vi "TEST PICOSCOPE 3000.vi"() -> ()   [LabVIEW 2018]
panel:
  in  "Acquisition Settings":T1={"preTriggerSamples"=0, "postTriggerSamples"=10000, "timebase"=5000, "Down-Sample Mode"=0, "Down Sample Ratio"=1} {"Down Sample Ratio" min=1 step=1; "Down-Sample Mode" items=["None"=0, "Aggregate"=1, "Decimate"=2, "Average"=4]; "postTriggerSamples" max=10000 step=100}
  out "Device Info":T2
  in  "Channel B Settings":T3={"Enabled"=TRUE, "Coupling"=1, "Range"=6, "Analogue Offset"=0.0} {"Range" items=["20 mV"=1, "50 mV"=2, "100 mV"=3, "200 mV"=4, "500 mV"=5, "1 V"=6, "2 V"=7, "5 V"=8, "10 V"=9, "20 V"=10]; "Coupling" items=["AC", "DC"]}
  in  "Channel A Settings":T3={"Enabled"=TRUE, "Coupling"=1, "Range"=6, "Analogue Offset"=0.0} {"Range" items=["20 mV"=1, "50 mV"=2, "100 mV"=3, "200 mV"=4, "500 mV"=5, "1 V"=6, "2 V"=7, "5 V"=8, "10 V"=9, "20 V"=10]; "Coupling" items=["AC", "DC"]}
  out "Waveform Graph 2":T4(graph)
  out "Waveform Graph":T4(graph)
  in  "Trigger Settings":T5={"Trigger Enabled"=TRUE, "Trigger Source"=enum."Channel A", "Trigger Threshold (Volts)"=0.0, "Trigger Direction"=2, "Trigger Delay (samples)"=0, "Auto Trigger Time (ms)"=1000} {"Trigger Direction" items=["Rising"=2, "Falling"=3]}
  # "127"
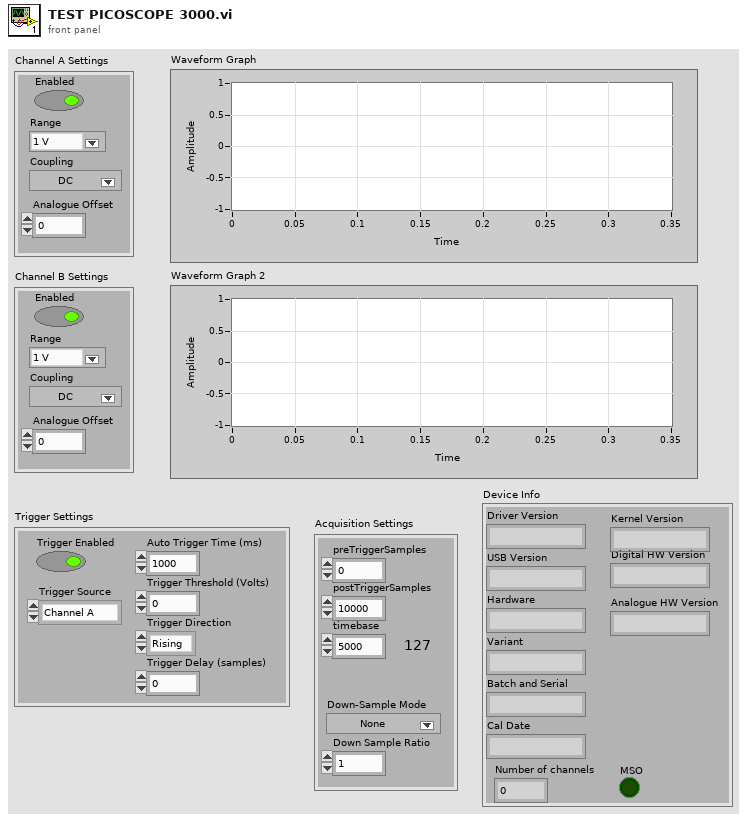
[diagram p1: front panel]
types:
  T1 = cluster{"preTriggerSamples":u32, "postTriggerSamples":u32, "timebase":u32, "Down-Sample Mode":i32, "Down Sample Ratio":u32}
  T2 = cluster{"Driver Version":string, "USB Version":string, "Hardware":string, "Variant":string, "Batch and Serial":string, "Cal Date":string, "Kernel Version":string, "Digital HW Version":string, "Analogue HW Version":string, "MSO":bool, "Number of channels":i16}
  T3 = cluster{"Enabled":bool, "Coupling":i16, "Range":u16, "Analogue Offset":sgl}
  T4 = cluster{i32, "Sample Internal":sgl, "Data (Volts)":dbl[]}
  T5 = cluster{"Trigger Enabled":bool, "Trigger Source":enum16{"Channel A", "Channel B", "Channel C", "Channel D", "Ext."}, "Trigger Threshold (Volts)":dbl, "Trigger Direction":u16, "Trigger Delay (samples)":u32, "Auto Trigger Time (ms)":i16}
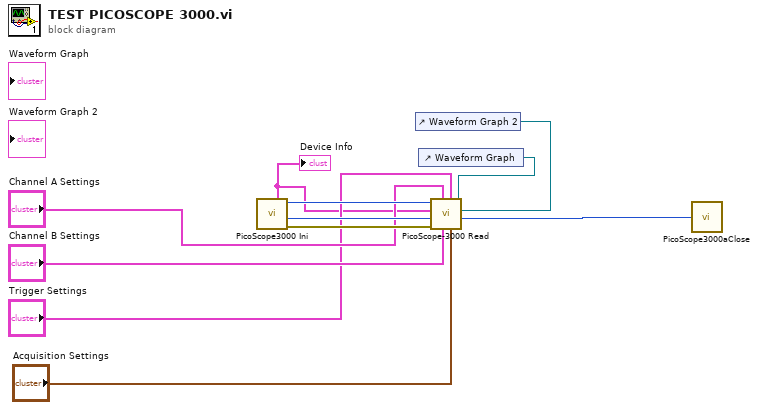
[diagram p0: block diagram]
diagram:
  n1 = call "PicoScope3000 Ini.vi"() -> ("error out"=w6:errorcluster, "Max Adc value"=w7:i16, "handle"=w11:i16, "Device Info"=w1:T2)  [unwired: 6 in, 2 out]
  "Device Info" <- w1
  n2 = control-ref of="Waveform Graph 2"() -> (w8:refnum<vi>)
  n3 = control-ref of="Waveform Graph"() -> (w9:refnum<vi>)
  n4 = call "PicoScope-3000 Read.vi"("WFD-Ref Ch-B"=w8, "WFD-Ref Ch-A"=w9, "Acquisition Settings"="Acquisition Settings", "Trigger Settings"="Trigger Settings", "Channel B Settings"="Channel B Settings", "Channel A Settings"="Channel A Settings", "error in"=w6, "Max Adc value"=w7, "Device Info"=w1, "handle"=w11) -> ("handle"=w10:i16)  [unwired: 1 out]
  n5 = call "PicoScope3000aClose.vi"("handle"=w10) -> ()
